vi "Corr Transducers Edit Panel.vi"(8 "error in":errorcluster, 11 "path corr":path caption="Correction file path") -> (0 "error out":errorcluster, 3 "path corr out":path caption="Correction file path")   [LabVIEW 2013]
uses:
  Corr Transducer INFO Item.ctl
  Corr Transducer INFO Record.ctl
  varilib/varilib.lvlib
panel:
  out "items":T1[](array[typedef])
  in  "btn save":bool
  in  "Type":string
  in  "btn ok":bool
  in  "btn csv":bool
  in  "CSV table path (relative)":string
  in  "Uncertainty":dbl format="%#_8p"
  in  "Value":dbl format="%#_8p"
  in  "Digitizer channel identifier (optional)":string
  in  "Serial number":string
  in  "Name":string
  in  "Correction item":u16(ring) items=["nominal ratio", "amplitude transfer path", "phase transfer path", "rvd low side impedance path", "output terminals series impedance path", "output terminals series impedance path (low-side)", "output terminals mutual inductance path", "output terminals shunting admittance path", "output cable series impedance path", "output cable shunting admittance path", "buffer output series impedance path"]
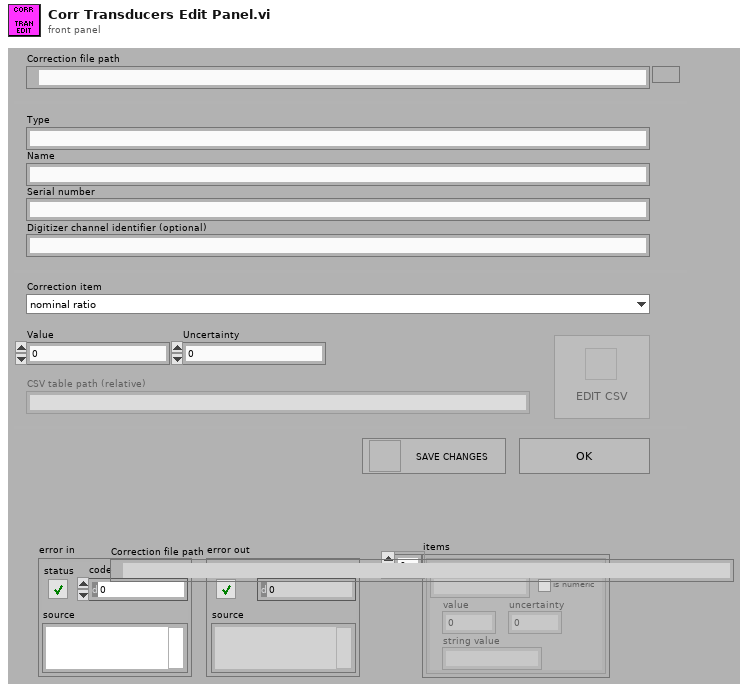
[diagram p1: front panel]
types:
  T1 = typedef "Corr Transducer INFO Item.ctl" = cluster{"name":string, "is numeric":bool, "value":dbl, "uncertainty":dbl, "string value":string}
  T2 = typedef "Corr Transducer INFO Record.ctl" = cluster{"name":string, "serial":string, "channel name":string, "items":T1[], "type":string}
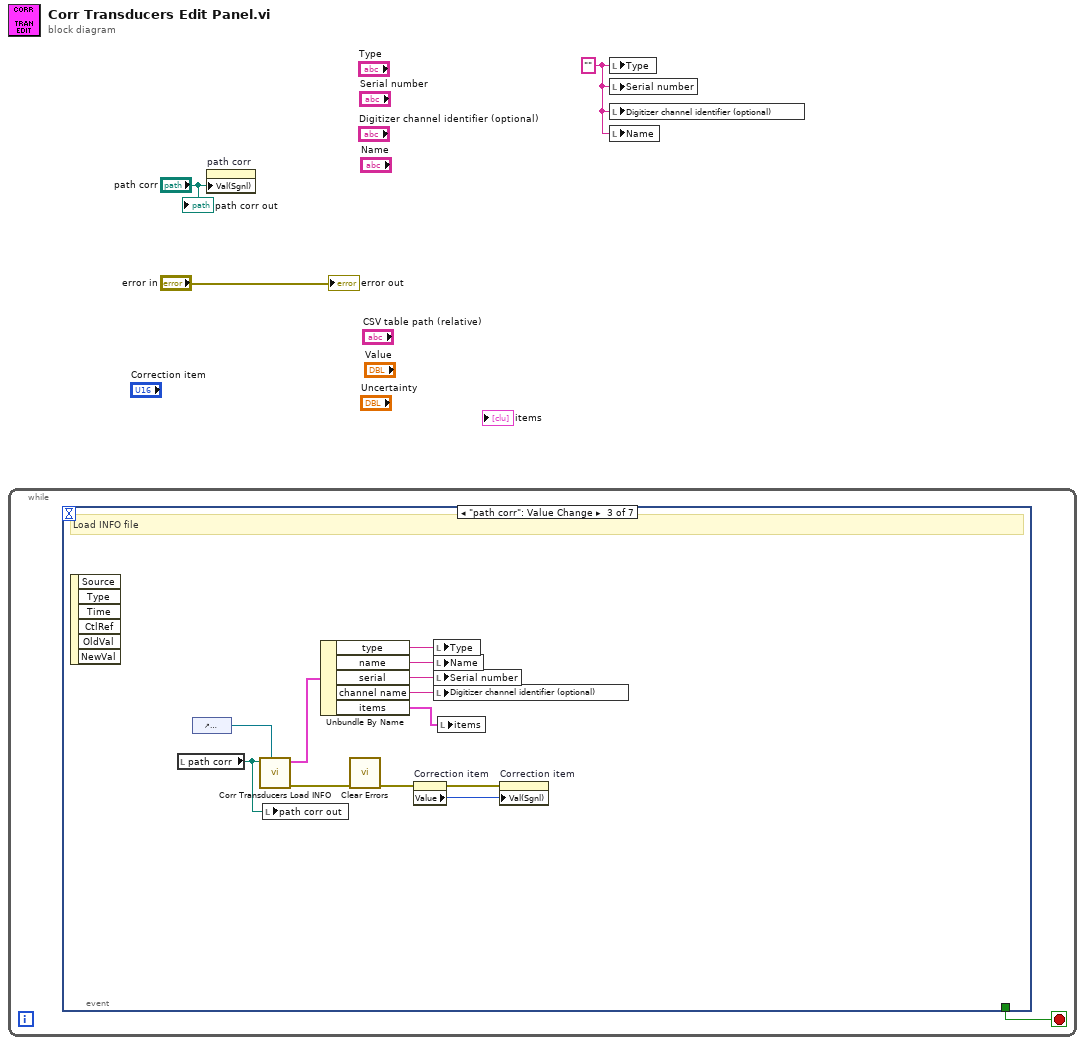
[diagram p0: block diagram]
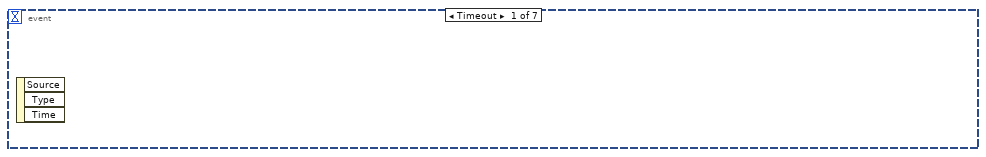
[diagram p2: hidden frame]
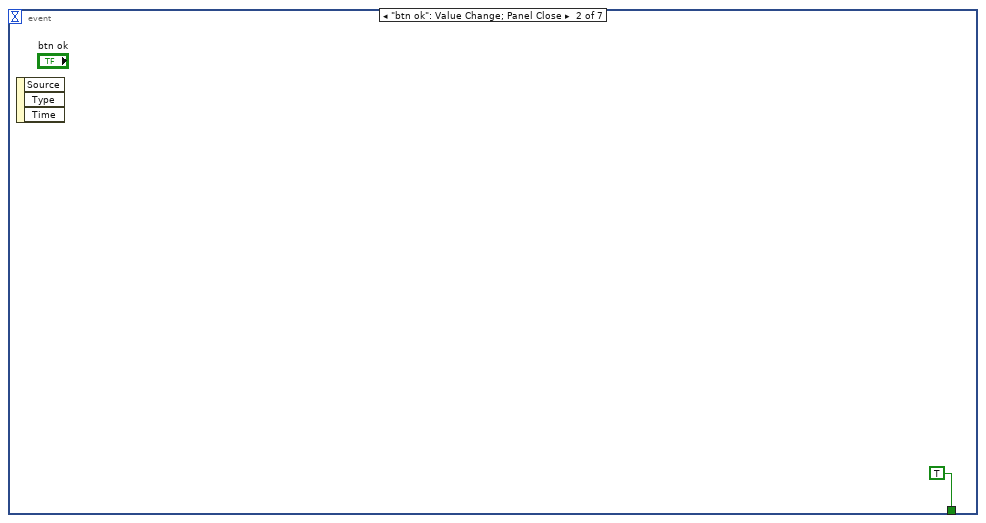
[diagram p3: hidden frame]
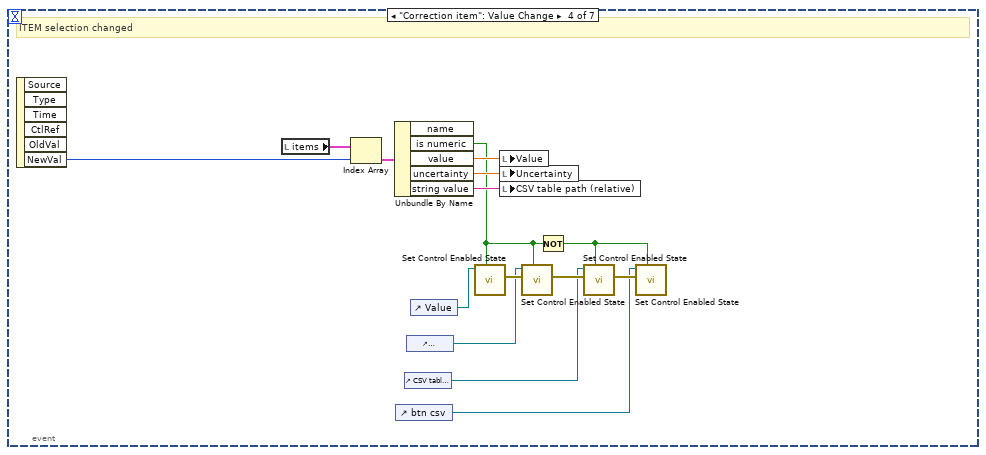
[diagram p4: hidden frame]
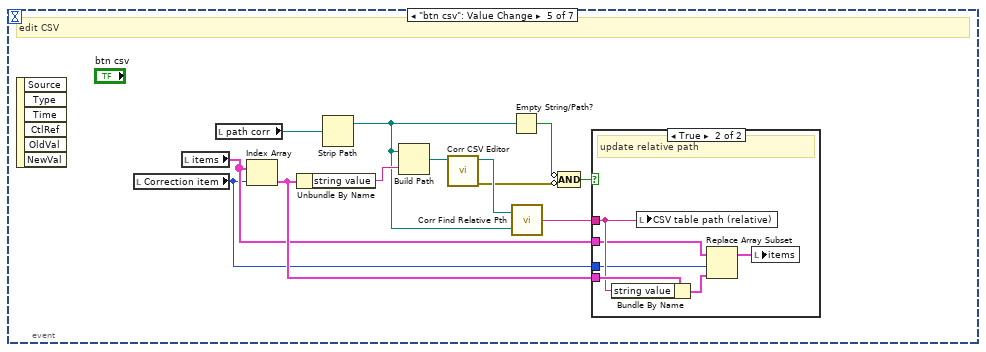
[diagram p5: hidden frame]
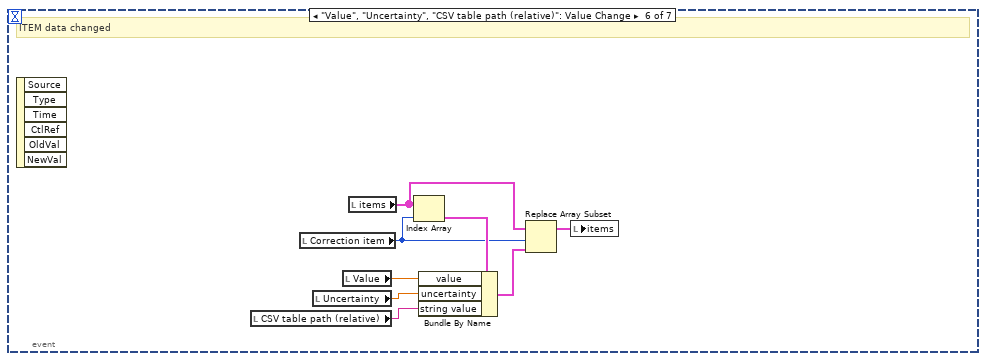
[diagram p7: hidden frame]
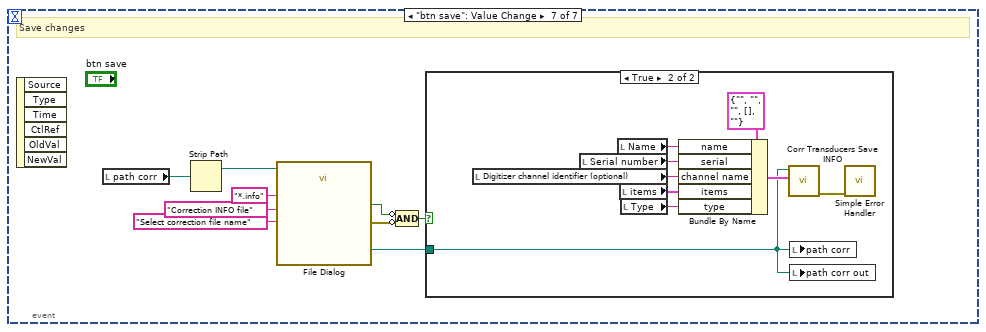
[diagram p8: hidden frame]
diagram:
  w1 = "" ("Type")
  n1 = while {
    stop <- w4 stop-if-true
    n2 = event shown="[2] \"path corr\": Value Change" {
      selector: _ -> [_ _ _ _ _ _ _]
      dyn-events: _ -> [_ _ _ _ _ _ _]
      timeout: _ -> [_ _ _ _ _ _ _]
      tunnel: [_ TRUE _ _ _ _ _] -> w4
      event Timeout {
        n3 = event-data() -> ()  [unwired: 1 in, 3 out]
      }
      event "btn ok": Value Change; Panel Close {
        n4 = event-data() -> ()  [unwired: 1 in, 3 out]
      }
      event "path corr": Value Change {
        # "Load INFO file"
        n5 = event-data() -> ()  [unwired: 1 in, 6 out]
        n6 = local read "path corr"() -> (w6:path)
        n7 = control-ref of="Correction item"() -> (w11:refnum<vi>)
        n8 = call "Corr Transducers Load INFO.vi"("item ref"=w11, "Path"=w6) -> ("error out"=w17:errorcluster, "transducer info"=w16:T2)  [unwired: 8 in]
        n9 = local write "path corr out"(w6) -> ()
        n10 = Unbundle By Name(w16) -> ("type"=w15:string, "name"=w14:string, "serial"=w13:string, "channel name"=w12:string, "items"=w7:T1[])
        n11 = call <vilib>:"Clear Errors.vi"("error in (no error)"=w17) -> ("error out"=w10:errorcluster)  [unwired: 6 in]
        n12 = property on="Correction item" class="Ring (strict)"(error in=w10) -> (error out=w9:errorcluster, "Value"=w8:u16)  [unwired: 1 in, 1 out]
        n13 = local write "Type"(w15) -> ()
        n14 = local write "Name"(w14) -> ()
        n15 = local write "Serial number"(w13) -> ()
        n16 = local write "Digitizer channel identifier (optional)"(w12) -> ()
        n17 = local write "items"(w7) -> ()
        n18 = property on="Correction item" class="Ring (strict)"(error in=w9, "Val(Sgnl)"=w8) -> ()  [unwired: 1 in, 2 out]
      }
      event "Correction item": Value Change {
        # "ITEM selection changed"
        n19 = event-data() -> ("NewVal"=w32:u16)  [unwired: 1 in, 5 out]
        n20 = local read "items"() -> (w18:T1[])
        n21 = Index Array(array=w18, index=w32) -> (element=w31:T1)
        n22 = Unbundle By Name(w31) -> ("is numeric"=w26:bool, "value"=w30:dbl, "uncertainty"=w29:dbl, "string value"=w28:string)  [unwired: 1 out]
        n23 = control-ref of="btn csv"() -> (w19:refnum<vi>)
        n24 = control-ref of="CSV table path (relative)"() -> (w22:refnum<vi>)
        n25 = control-ref of="Uncertainty"() -> (w24:refnum<vi>)
        n26 = control-ref of="Value"() -> (w25:refnum<vi>)
        n27 = call "Set Control Enabled State.vi"("enabled (T)"=w26, "reference in"=w25) -> ("error out"=w27:errorcluster)  [unwired: 8 in, 1 out]
        n28 = local write "Value"(w30) -> ()
        n29 = local write "Uncertainty"(w29) -> ()
        n30 = local write "CSV table path (relative)"(w28) -> ()
        n31 = call "Set Control Enabled State.vi"("enabled (T)"=w26, "error in (no error)"=w27, "reference in"=w24) -> ("error out"=w23:errorcluster)  [unwired: 7 in, 1 out]
        n32 = Not(x=w26) -> (.not. x?=w20:bool)
        n33 = call "Set Control Enabled State.vi"("enabled (T)"=w20, "error in (no error)"=w23, "reference in"=w22) -> ("error out"=w21:errorcluster)  [unwired: 7 in, 1 out]
        n34 = call "Set Control Enabled State.vi"("enabled (T)"=w20, "error in (no error)"=w21, "reference in"=w19) -> ()  [unwired: 7 in, 2 out]
      }
      event "btn csv": Value Change {
        # "edit CSV"
        n35 = event-data() -> ()  [unwired: 1 in, 6 out]
        n36 = local read "Correction item"() -> (w33:u16)
        n37 = local read "items"() -> (w34:T1[])
        n38 = local read "path corr"() -> (w41:path)
        n39 = Index Array(array=w34, index=w33) -> (element=w35:T1)
        n40 = Unbundle By Name(w35) -> ("string value"=w44:string)
        n41 = Strip Path(path=w41) -> (stripped path=w36:path)  [unwired: 1 out]
        n42 = Build Path(base path=w36, name or relative path=w44) -> (appended path=w43:path)
        n43 = call "Corr CSV Editor.vi"("File path"=w43) -> ("error out"=w39:errorcluster, "path out"=w42:path)  [unwired: 9 in]
        n44 = Empty String/Path?(string/path=w36) -> (empty?=w40:bool)
        n45 = call "Corr Find Relative Pth.vi"("INFO path"=w36, "CSV path"=w42) -> ("CSV relative path"=w37:string)
        n46 = Compound Arithmetic op=AND(invert w40, invert w39) -> (w38:bool)
        n47 = case shown="True" w38 {
          tunnel: w37 -> [_ w49]
          tunnel: w35 -> [_ w50]
          tunnel: w34 -> [_ w48]
          tunnel: w33 -> [_ w46]
          frame False {
          }
          frame True {
            # "update relative path"
            n48 = Bundle By Name(cluster=w50, "string value"=w49) -> (w47:T1)
            n49 = local write "CSV table path (relative)"(w49) -> ()
            n50 = Replace Array Subset(array=w48, new element=w47, index=w46) -> (w45:T1[])
            n51 = local write "items"(w45) -> ()
          }
        }
      }
      event "Value", "Uncertainty", "CSV table path (relative)": Value Change {
        # "ITEM data changed"
        n52 = event-data() -> ()  [unwired: 1 in, 6 out]
        n53 = local read "CSV table path (relative)"() -> (w55:string)
        n54 = local read "Correction item"() -> (w53:u16)
        n55 = local read "Uncertainty"() -> (w56:dbl)
        n56 = local read "Value"() -> (w57:dbl)
        n57 = local read "items"() -> (w54:T1[])
        n58 = Index Array(array=w54, index=w53) -> (element=w58:T1)
        n59 = Bundle By Name(cluster=w58, "value"=w57, "uncertainty"=w56, "string value"=w55) -> (w52:T1)
        n60 = Replace Array Subset(array=w54, new element=w52, index=w53) -> (w51:T1[])
        n61 = local write "items"(w51) -> ()
      }
      event "btn save": Value Change {
        # "Save changes"
        n62 = event-data() -> ()  [unwired: 1 in, 6 out]
        n63 = local read "path corr"() -> (w67:path)
        n64 = Strip Path(path=w67) -> (stripped path=w66:path)  [unwired: 1 out]
        n65 = call "File Dialog"("start path"=w66, "prompt"="Select correction file name", "pattern (all files)"="*.info", "pattern label"="Correction INFO file") -> ("selected path"=w59:path, "cancelled"=w61:bool, "error out"=w62:errorcluster)  [unwired: 8 in, 1 out]
        n66 = Compound Arithmetic op=AND(invert w61, invert w62) -> (w60:bool)
        n67 = case shown="True" w60 {
          tunnel: w59 -> [_ w68]
          frame False {
          }
          frame True {
            n68 = local read "Digitizer channel identifier (optional)"() -> (w69:string)
            n69 = local read "Serial number"() -> (w71:string)
            n70 = local read "Name"() -> (w70:string)
            n71 = local read "items"() -> (w73:T1[])
            n72 = local read "Type"() -> (w72:string)
            n73 = Bundle By Name(cluster=T2 {"name"="", "serial"="", "channel name"="", "items"=[], "type"=""} ("transducer info"), "name"=w70, "serial"=w71, "channel name"=w69, "items"=w73, "type"=w72) -> (w74:T2)
            n74 = call "Corr Transducers Save INFO.vi"("transducer info"=w74, "Path"=w68) -> ("error out"=w76:errorcluster)  [unwired: 9 in]
            n75 = local write "path corr"(w68) -> ()
            n76 = local write "path corr out"(w68) -> ()
            n77 = call <vilib>:"Simple Error Handler.vi"("error in (no error)"=w76) -> ()  [unwired: 4 in, 5 out]
          }
        }
      }
    }
  }
  n78 = property on="path corr" class="Path"("Val(Sgnl)"="path corr") -> ()  [unwired: 2 in, 2 out]
  n79 = local write "Type"(w1) -> ()
  n80 = local write "Serial number"(w1) -> ()
  n81 = local write "Digitizer channel identifier (optional)"(w1) -> ()
  n82 = local write "Name"(w1) -> ()
  "error out" <- "error in"
  "path corr out" <- "path corr"
